vi "Main-revision3.vi"() -> ()   [LabVIEW 2013]
uses:
  Controls/GUI controls/TabControl--Tab.ctl
  Controls/Loop_data--Cluster.ctl
  Controls/Graph_data--Cluster.ctl
  Controls/GUI controls/GUI_Flags.ctl
  Shared/MySQL/typedefs/mysql_authentication.ctl
  Controls/Database Data.ctl
  Shared/MySQL/Preset Query Enum.ctl
  <userlib>/_OpenG.lib/array/array.llb/Filter 1D Array with Scalar (String)__ogtk.vi
panel:
  out "chnl data":string[](array[string])
  out "channels":string[](array[string])
  out "Selected Variables":string[][](array[string])=[["LB_EnergyMeter_1", "Reading.Channel 1", "Preamp [mJ]", "", "", ""], ["LB_EnergyMeter_2", "Reading.Channel 1", "Amplifier 2 [J]", "", "", ""], ["HPD_CCD", "exposure", "exposure", "0.003", "0.08", "0.0003"]]
  out "Device Infor from Database":string[][](array[string])
  out "subscribe messages\nfor Device status":string[](array[string])
  out "tcp Data":string[][](array[string])=[["LB_EnergyMeter_1 LB_EnergyMeter_1 shot #", "LB_EnergyMeter_1 reading.channel 1", "LB_EnergyMeter_2 LB_EnergyMeter_2 shot #", "LB_EnergyMeter_2 reading.channel 1", "HPD_CCD HPD_CCD shot #", "HPD_CCD exposure"], ["0", "0.029234726", "0", "0.000000000", "0", "0.003000"]]
  in  "Tab Control":enum32{"Home", "Settings", "Plot", "Save"}(tab)
  in  "Database Variable List":i32[](listbox)
  in  "Plotter ID (Simulate)":string
  out "Query":string
  in  "Add variables":bool
  out "Long Term Plot":cluster{timestamp[], dbl[]}[](graph)
  in  "Clear Graph":bool
  out "short Term Plot":cluster{timestamp[], dbl[]}[](graph) caption="Long Term Plot"
  in  "Stop":bool
  in  "Simulate":bool
  out "appargs 2":string[](array[string])
  out "min Left":i16
  out "min Top":i16
  out "max Right":i16
  out "max Bottom":i16
  in  "Read INI File":bool
  in  "Configuration File Path":path=path "C:/Users/Priyanka/Documents/Plotter/Data/Plot Configuration.txt"
  out "Subscribe commands":string[](array[string])=["Wait>>Exposure,Gain", "Wait>>Exposure"]
  out "appended array":string[][](array[string])
  in  "Plot":bool=TRUE
  in  "Settings":bool
  in  "Home":bool
  # "Settings"
  # "Plot"
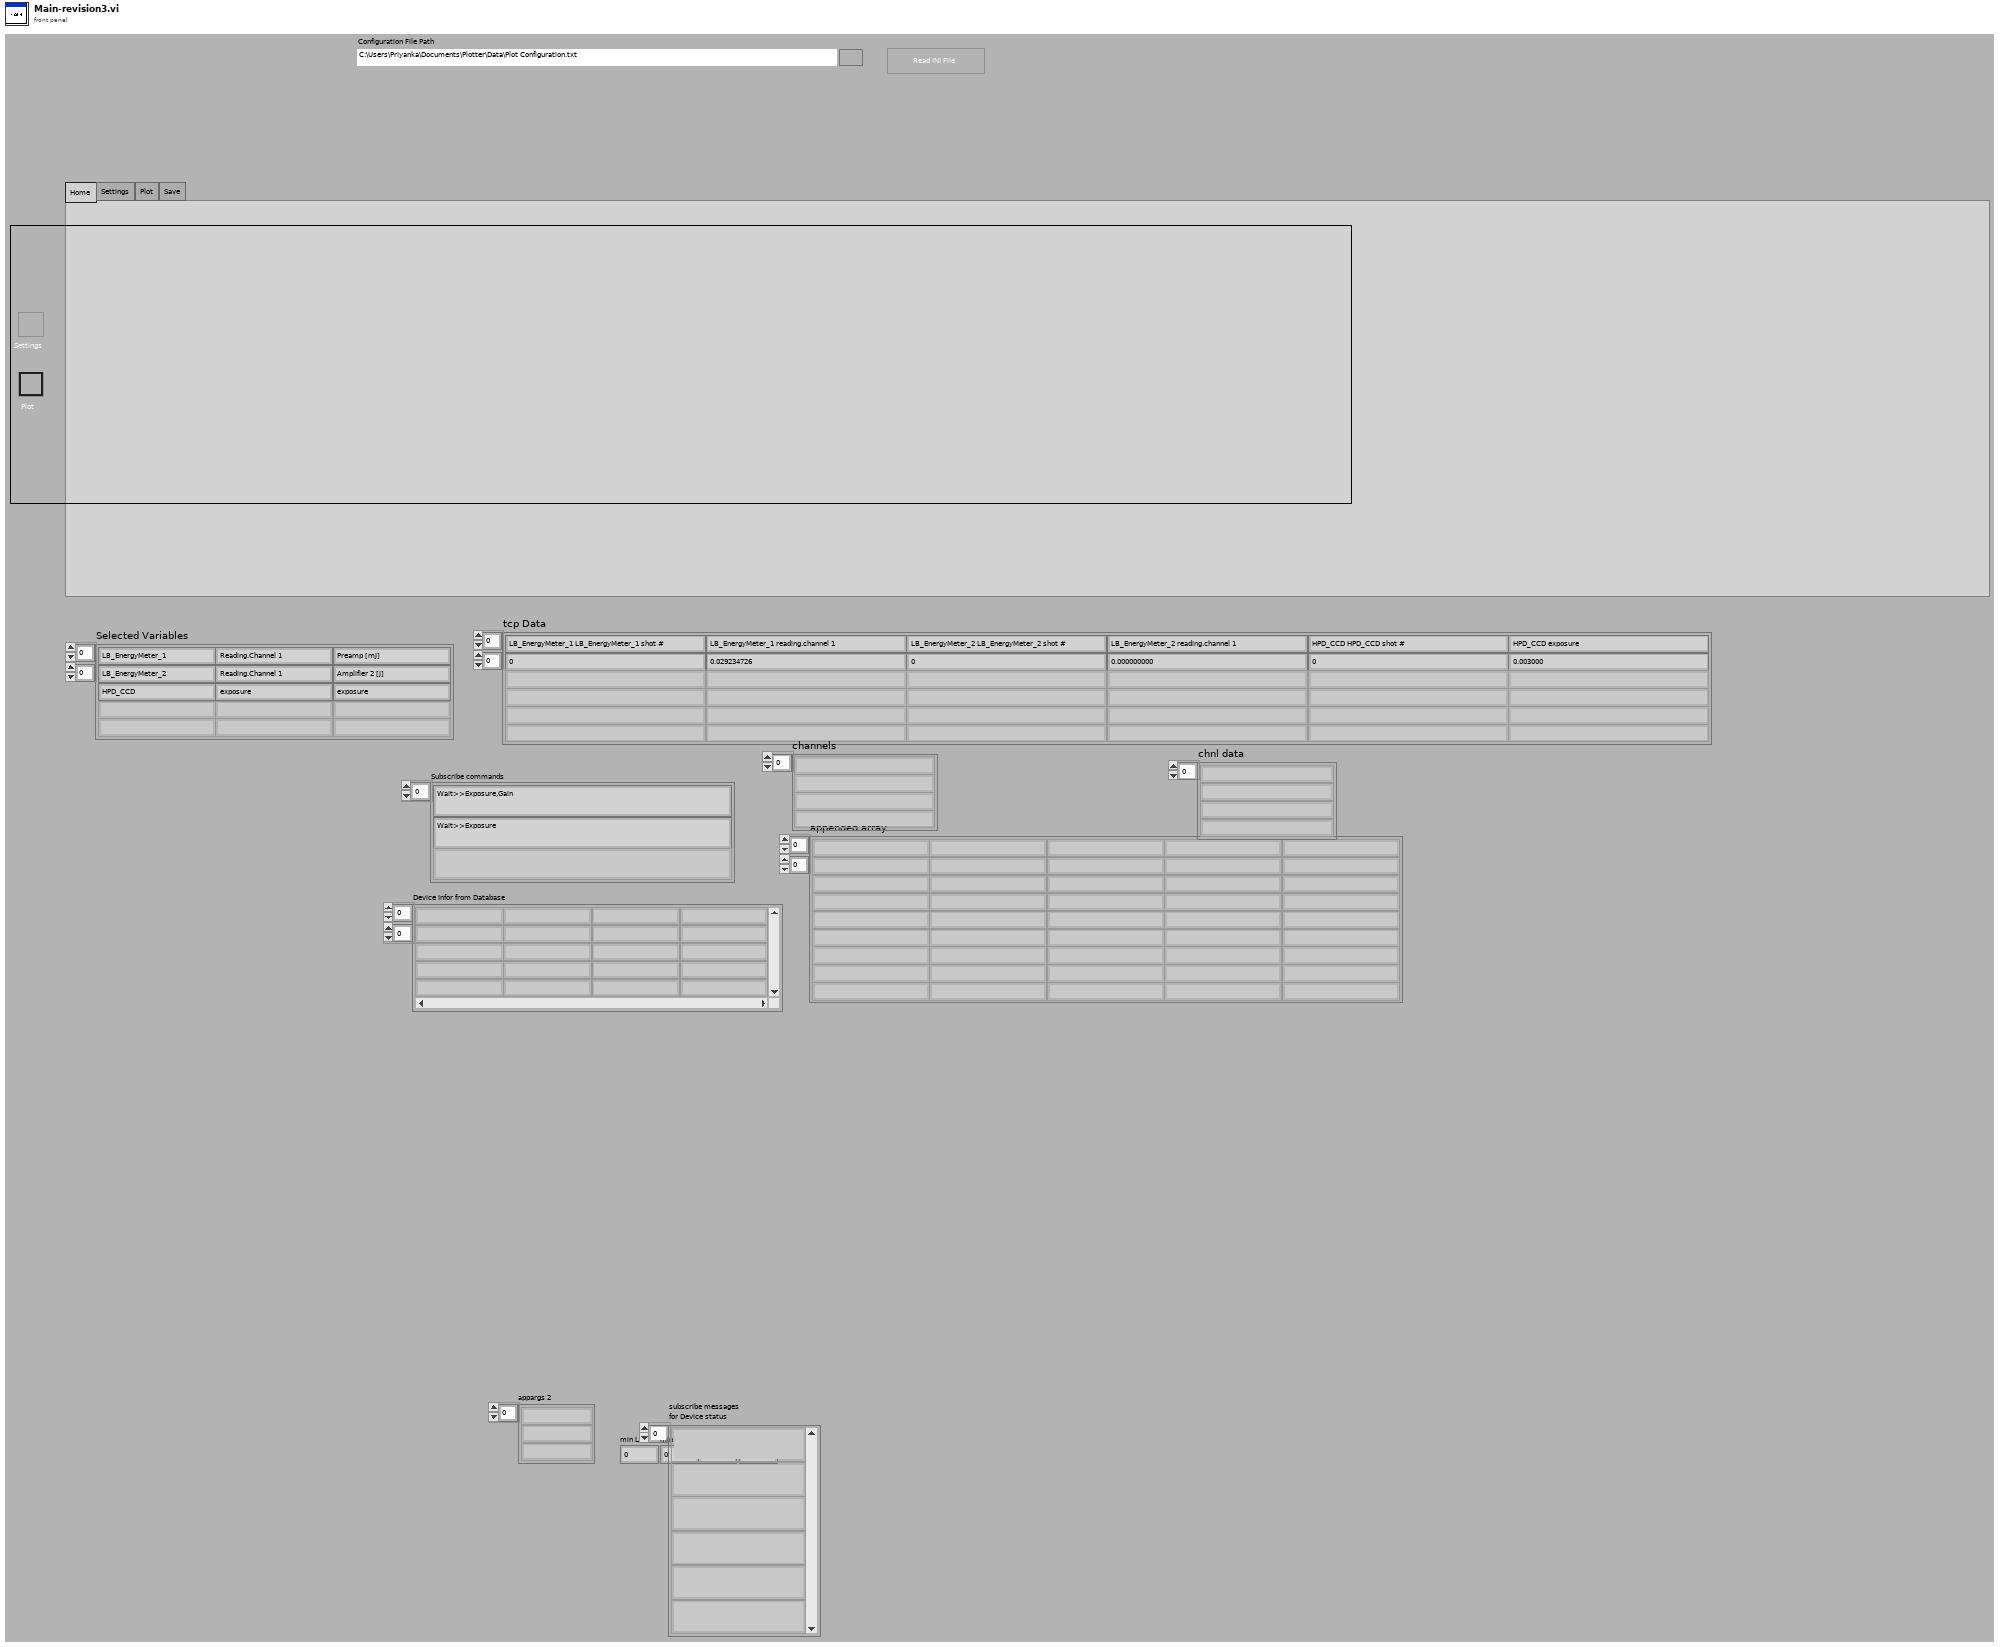
[diagram p1: front panel]
types:
  T1 = typedef "Preset Query Enum.ctl" = enum16{"Get Locations", "Get all IPs and MACs", "Get classes", "Get expt variables to set at scanstart for particular device", "Get expt devices and variables with start values", "Get expt devices and variables (with data to get)", "Get expt devices with data to get", "Get Expt devices and GUIs", "Get all devices basic properties", "Get Virtual Devices Core Info", "Get Expt names", "Get experiment basic properties", "Get experiment alarm variables", "Get MC Ports", "Get device network comm port", "Get devicetype lvclass path", "Get basic device properties", "Get Init Order", "Get all setable variables of a device", "Get device variable aliases", "Get force values of all settable variables", "Get all variables of a devicetype", "Get all variables of a device", "Get plotter details", "Get Saved Scans", "Get Scan Info", "GetGeneralGUIs", "Get expt for plotter", "Get plotter IDs from expt", "Get all devices", "Get all Virtual Devices", "Get all aliases", "Get variable and device info for Virtual Device", "GetItemLocatorIP", "Get IPs for GUIs", "Get DeviceType from Device", "GetLocalPortRange", "GetDevicePresetVariables", "Get Device Configuration", "GetAllPresetNames", "GetAllConfigurationNames", "GetPresetDeviceNames"}
  T2 = typedef "LVAllMonitorsDisplayTypeDef.ctl" = cluster{"Bounds":cluster{"Left":i16, "Top":i16, "Right":i16, "Bottom":i16}, "Depth":i16}[]
  T3 = typedef "tcp_new_data_event.ctl" = refnum<user-event>
  T4 = typedef "TabControl--Tab.ctl" = enum32{"Home", "Settings", "Plot", "Save"}
  T5 = enum32{"invalid app kind", "Development System", "Run Time System", "Student Edition", "Embedded LabVIEW", "Evaluation", "Custom"}
  T6 = enum32{"Invalid", "Standard", "Closed", "Hidden", "Minimized", "Maximized"}
  T7 = typedef "Loop_data--Cluster.ctl" = cluster{"INI Data":string[][], "Currently selected items":i32[], "Selected Variables":string[][], "No of Selected Variables":i32, "Data":dbl[], "Simulate":bool, "Start":bool, "Legend Rows":i32, "Init":bool}
  T8 = typedef "Graph_data--Cluster.ctl" = cluster{"Graph Data Long":cluster{"Timestamp":timestamp[], "Data Array":dbl[]}[], "Graph Data Short":cluster{"Timestamp":timestamp[], "Data Array":dbl[]}[], "Short term plot":refnum<vi>, "Long term plot ":refnum<vi>, "ms timer value":u32}
  T9 = typedef "GUI_Flags.ctl" = cluster{"Start":bool, "Stop":bool, "Read INI File":bool, "Tab Control":enum32{"Home", "Settings", "Plot", "Save"}, "Settings":bool, "Home":bool, "Plot":bool}
  T10 = typedef "Database Data.ctl" = cluster{"SQL Server Info":cluster{"Port":u16, "IP Address":string, "Authentication":T11}, "Variables":string[], "Devices":string[], "Display Names (for variables)":string[], "Variable Data ID":string, "Variable display info":string[][], "Plotter ID":string, "Device space Variable":string[]}
  T11 = typedef "mysql_authentication.ctl" = cluster{"User":string, "Password":string, "Database":string}
  T12 = cluster{"Core":cluster{"Current VI Reference":refnum<vi>, "Close Panel on Exit?":bool}, "Data":T7, "Graph":T8, "GUI controls":T9, "PlotterInfo (from DB)":T10, "Subscribe commands":string[]}
  T13 = cluster{"Current VI Reference":refnum<vi>, "Close Panel on Exit?":bool}
  T14 = cluster{"Port":u16, "IP Address":string, "Authentication":T11}
  T15 = cluster{"Timestamp":timestamp[], "Data Array":dbl[]}[]
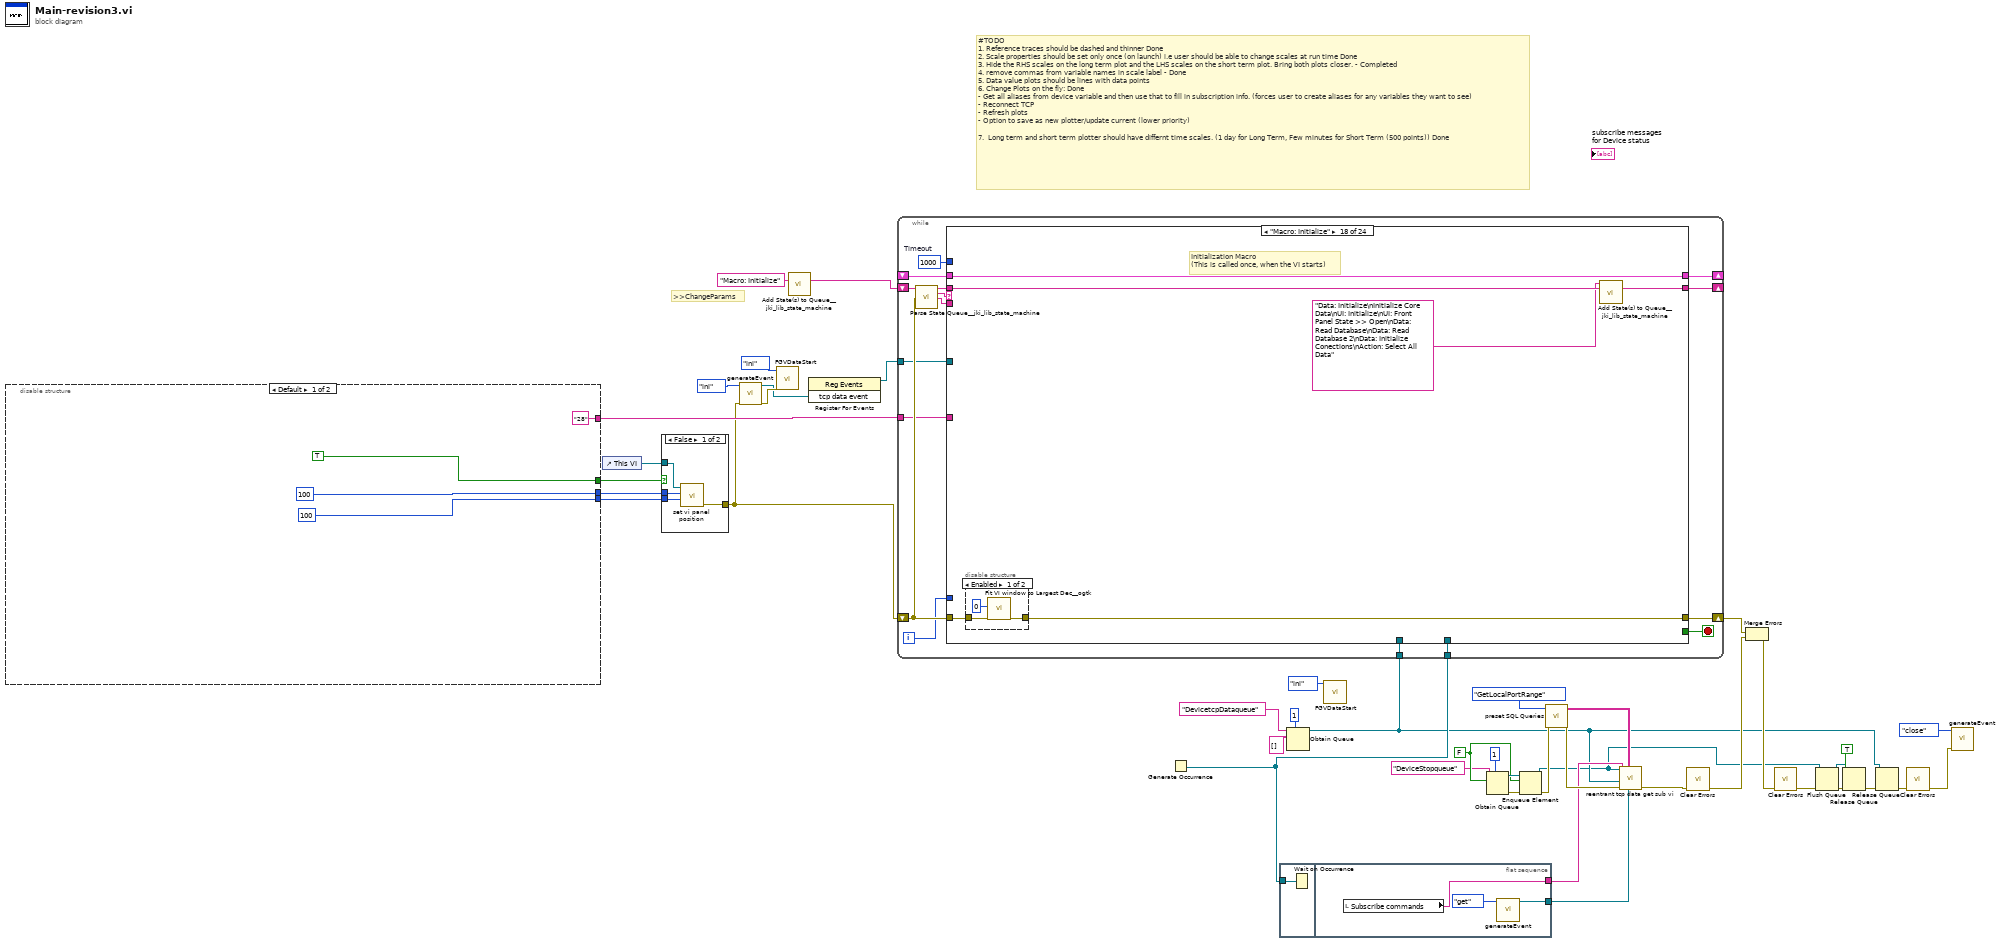
[diagram p0: block diagram]
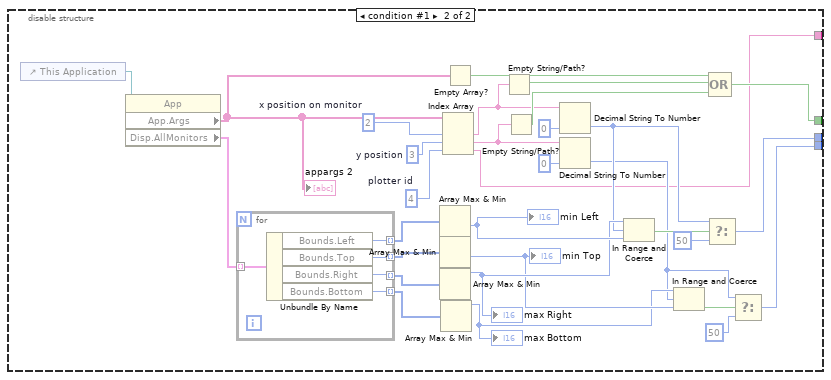
[diagram p3: hidden frame]
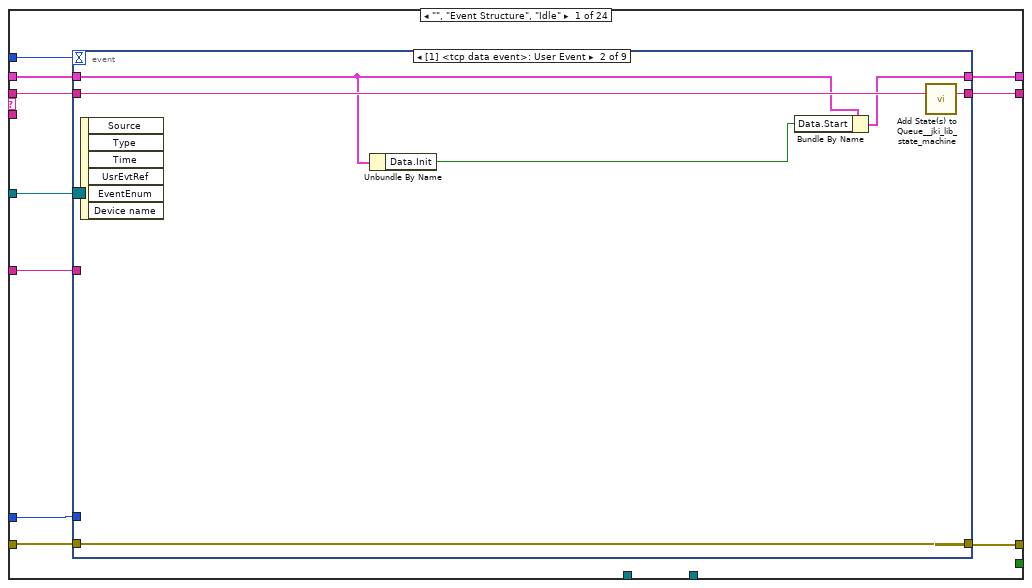
[diagram p4: hidden frame]
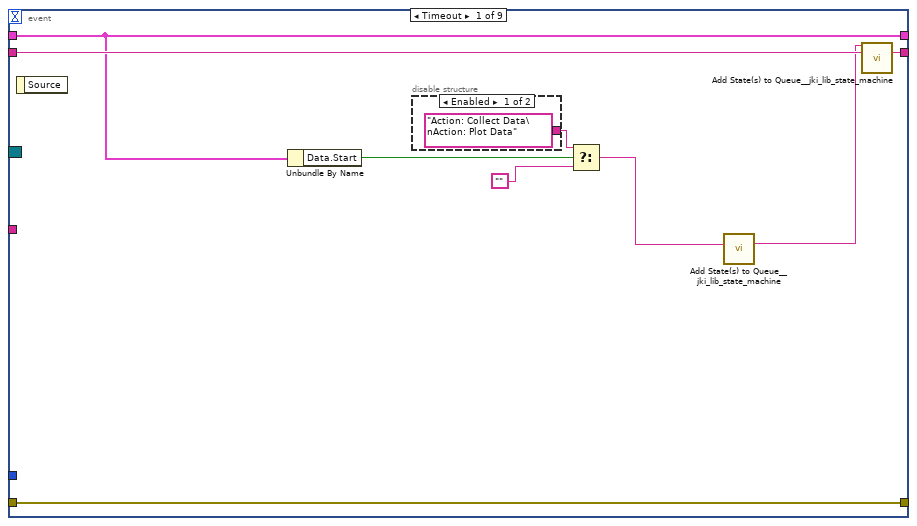
[diagram p5: hidden frame]
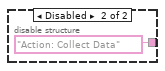
[diagram p6: hidden frame]
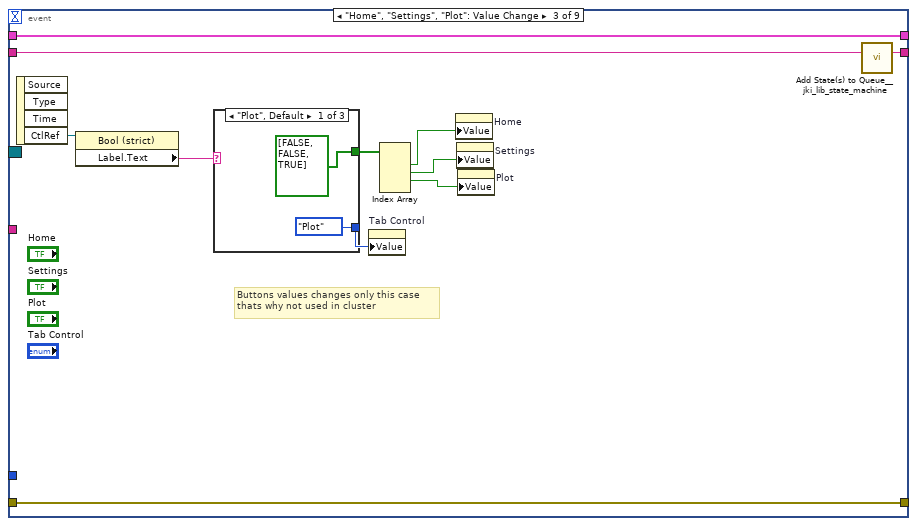
[diagram p7: hidden frame]
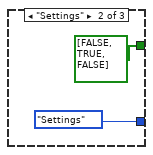
[diagram p8: hidden frame]
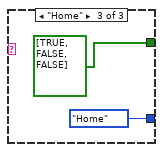
[diagram p9: hidden frame]
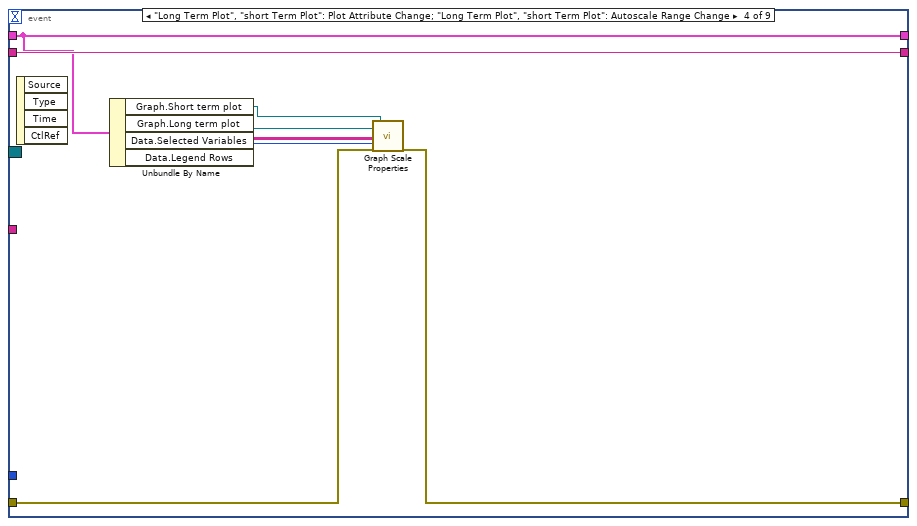
[diagram p10: hidden frame]
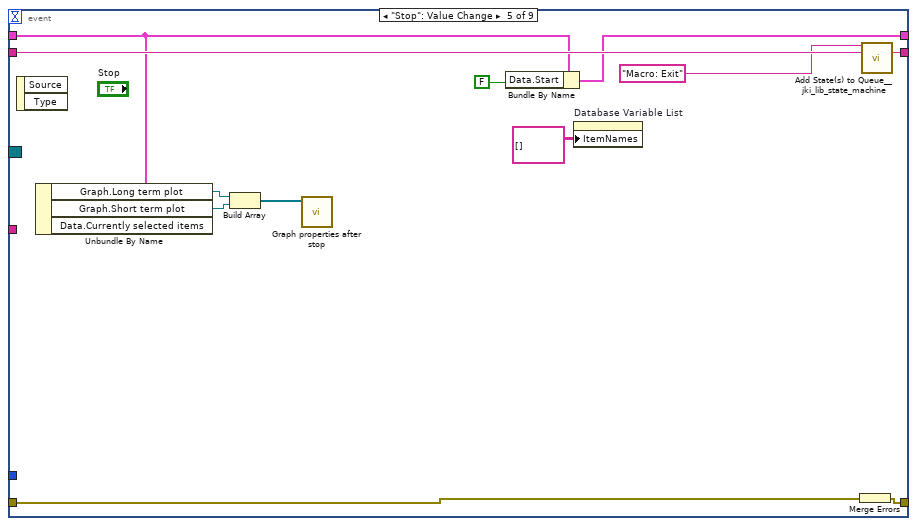
[diagram p11: hidden frame]
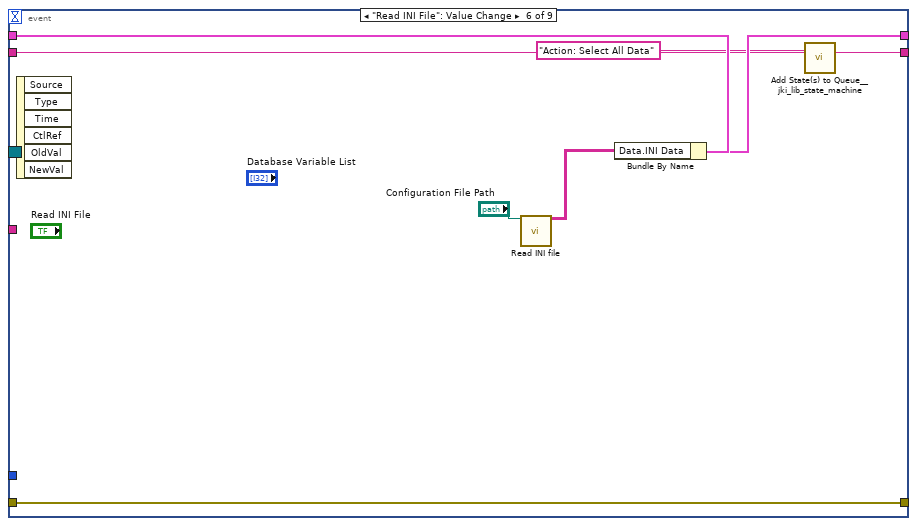
[diagram p12: hidden frame]
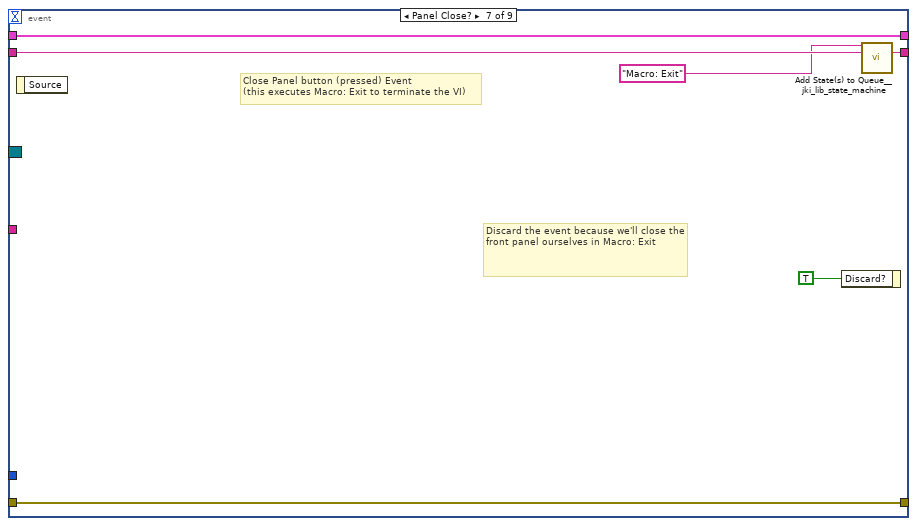
[diagram p13: hidden frame]
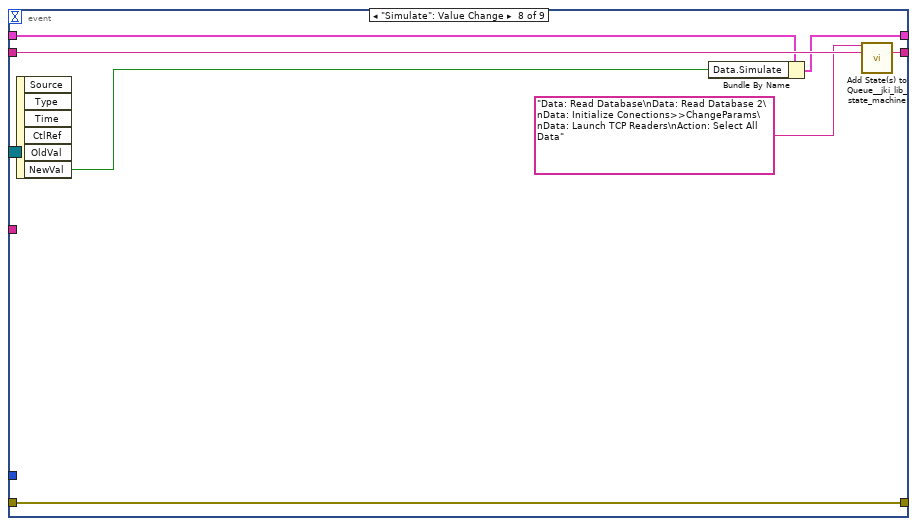
[diagram p14: hidden frame]
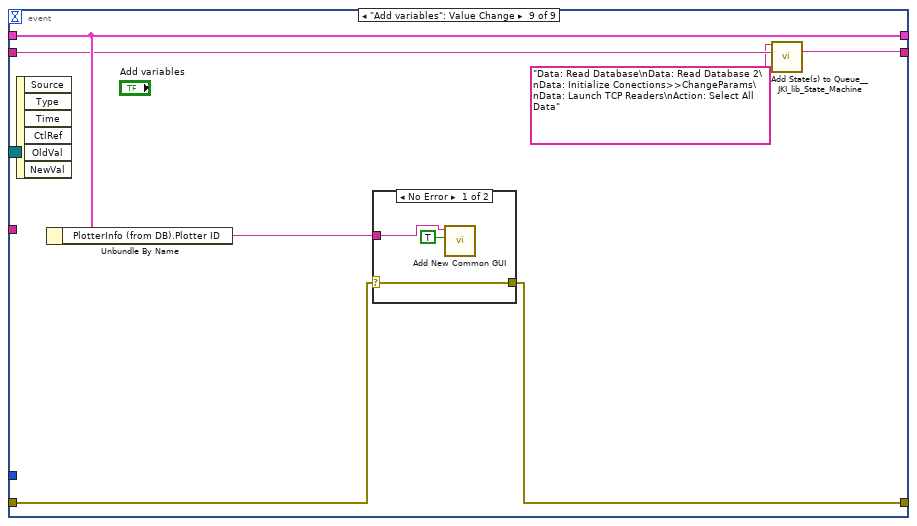
[diagram p15: hidden frame]
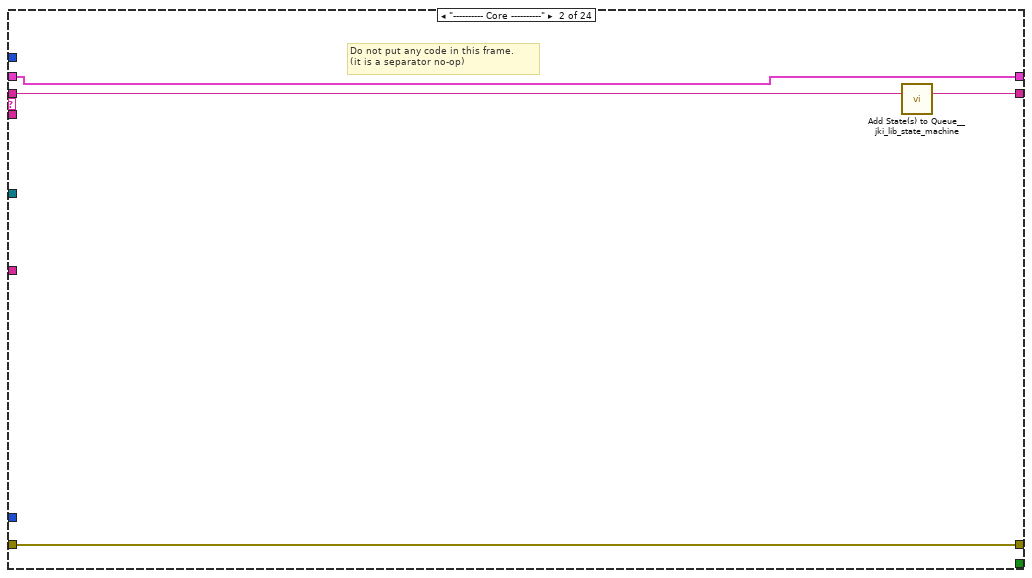
[diagram p17: hidden frame]
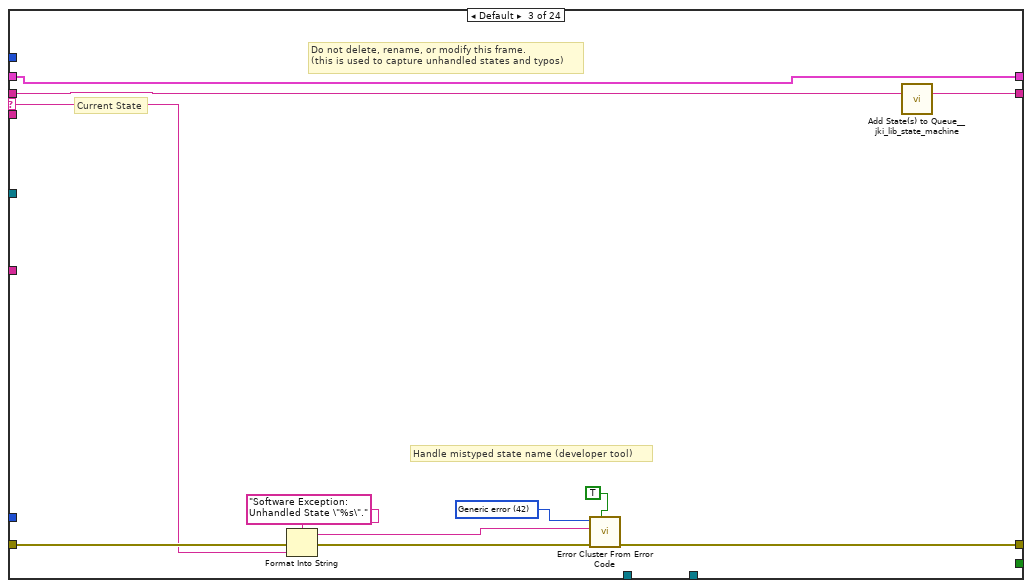
[diagram p18: hidden frame]
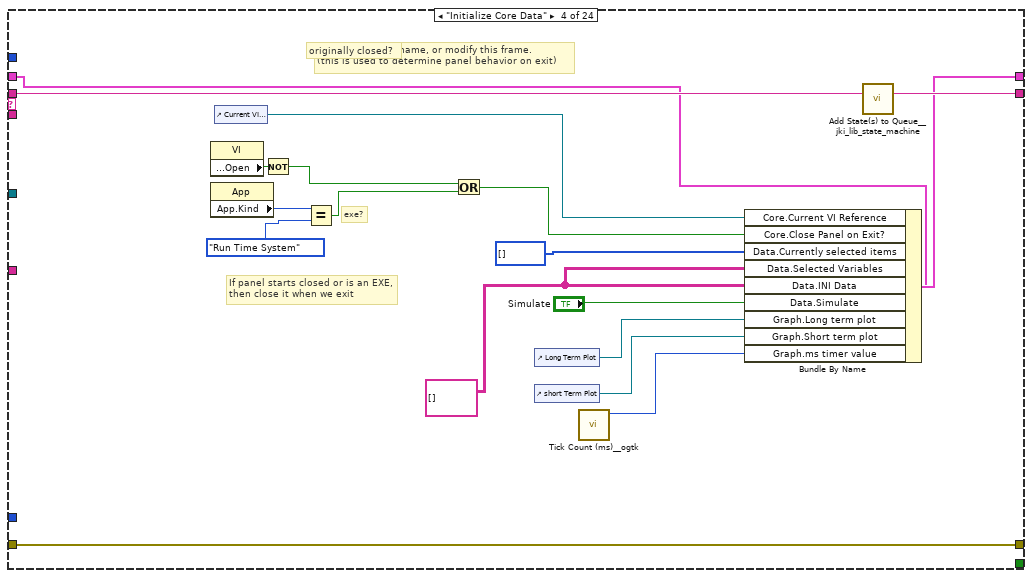
[diagram p19: hidden frame]
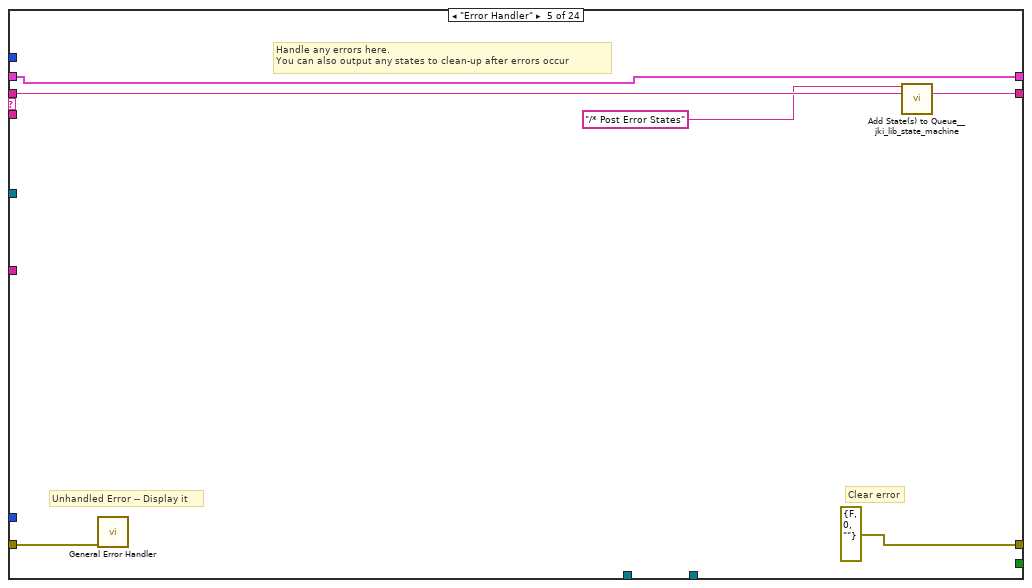
[diagram p20: hidden frame]
diagram:
  w23 = FALSE
  # ">>ChangeParams"
  # "#TODO\n1. Reference traces should be dashed and thinner Done\n2. Scale properties should be set only once (on launch) i.e user should be able to change scales at run time Done\n3. Hide the RHS scales on the long term plot and the LHS scales on the short term plot. Bring both plots closer. - Completed\n4. remove commas from variable names in scale label - Done \n5. Data value plots should be lines with data points\n6. Change Plots on the fly: Done\n- Get all aliases from device variable and then use that to fill in subscription info. (forces user to create aliases for any variables they want to see)\n- Reconnect TCP\n- Refresh plots\n- Option to save as new plotter/update current (lower priority)\n\n7.  Long term and short term plotter should have differnt time scales. (1 day for Long Term, Few minutes for Short Term (500 points)) Done"
  n1 = disable-structure shown="Default" {
    disable-tunnel: [100 ("number") w62] -> w39
    disable-tunnel: [100 ("number") w57] -> w40
    disable-tunnel: [TRUE w52] -> w41
    disable-tunnel: ["28" w49] -> w37
    frame condition #0 (active) {
    }
    frame condition #1 {
      w50 = 4  # plotter id
      w77 = 3  # y position
      w78 = 2  # x position on monitor
      n2 = control-ref of="This Application"() -> (w51:refnum<vi>)
      n3 = property class="App"(reference=w51) -> ("App.Args"=w76:string[], "Disp.AllMonitors"=w71:T2)  [unwired: 1 in, 2 out]
      "appargs 2" <- w76
      n4 = for {
        tunnel: w71 -> [w83] mode=indexing
        tunnel: [w82] -> w72 mode=indexing
        tunnel: [w81] -> w73 mode=indexing
        tunnel: [w80] -> w74 mode=indexing
        tunnel: [w79] -> w75 mode=indexing
        n5 = Unbundle By Name(w83) -> ("Bounds.Left"=w82:i16, "Bounds.Top"=w81:i16, "Bounds.Right"=w80:i16, "Bounds.Bottom"=w79:i16)
      }
      n6 = Array Max & Min(array=w72) -> (min value=w70:i16)  [unwired: 3 out]
      "min Left" <- w70
      n7 = Array Max & Min(array=w73) -> (min value=w68:i16)  [unwired: 3 out]
      "min Top" <- w68
      n8 = Array Max & Min(array=w74) -> (max value=w69:i16)  [unwired: 3 out]
      "max Right" <- w69
      n9 = Array Max & Min(array=w75) -> (max value=w67:i16)  [unwired: 3 out]
      "max Bottom" <- w67
      n10 = Index Array(array=w76, index #1=w78, index #2=w77, index #3=w50) -> (element #1=w48:string, element #2=w56:string, element #3=w49:string)
      n11 = Empty Array?(array=w76) -> (empty?=w55:bool)
      n12 = Empty String/Path?(string/path=w48) -> (empty?=w54:bool)
      n13 = Empty String/Path?(string/path=w56) -> (empty?=w53:bool)
      n14 = Decimal String To Number(string=w48, default (0L)=i16 0 ("default (0 I32)")) -> (number=w63:i16)  [unwired: 1 in, 1 out]
      n15 = Decimal String To Number(string=w56, default (0L)=i16 0 ("default (0 I32)")) -> (number=w58:i16)  [unwired: 1 in, 1 out]
      n16 = In Range and Coerce(upper limit=w69, x=w63, lower limit=w70) -> (In Range?=w64:bool)  [unwired: 1 out]
      n17 = In Range and Coerce(upper limit=w67, x=w58, lower limit=w68) -> (In Range?=w59:bool)  [unwired: 1 out]
      n18 = Select(t=w63, s=w64, f=i16 50) -> (s? t:f=w62:i16)
      n19 = Compound Arithmetic op=OR(w55, w54, w53) -> (w52:bool)
      n20 = Select(t=w58, s=w59, f=i16 50) -> (s? t:f=w57:i16)
    }
  }
  n21 = control-ref of="This VI"() -> (w38:refnum<vi>)
  n22 = case shown="False" w41 {
    tunnel: w39 -> [w87 _]
    tunnel: w40 -> [w86 _]
    tunnel: w38 -> [w85 _]
    tunnel: [w84 _] -> w6
    frame False {
      n23 = call "set vi panel position.vi"("top"=w86, "left"=w87, "This VI"=w85) -> ("error out"=w84:errorcluster)  [unwired: 7 in, 1 out]
    }
    frame True {
    }
  }
  n24 = call "generateEvent.vi"("error in"=w6, "command"=enum16{"ini", "get", "close"}."ini") -> ("error out"=w4:errorcluster, "tcp data event"=w2:T3)  [unwired: 8 in]
  n25 = call "FGVDataStart.vi"("error in"=w4, "command"=enum16{"ini", "get", "set"}."ini") -> ()  [unwired: 8 in, 2 out]
  n26 = call <vilib>:"Add State(s) to Queue__jki_lib_state_machine.vi"("State(s) in (\"\")"="Macro: Initialize") -> ("States Out"=w43:string)  [unwired: 14 in]
  n27 = register-events(w2) -> (reference out=w1:refnum<event-registration>)  [unwired: 2 in, 1 out]
  n28 = Generate Occurrence() -> (w15:refnum<k4>)
  n29 = flat-sequence {
    tunnel: w15 -> [w88]
    tunnel: [w89] -> w27
    tunnel: [w90] -> w28
    frame #0 {
      n30 = Wait on Occurrence(2:w88) -> ()  [unwired: 2 in, 1 out]
    }
    frame #1 {
      n31 = local read "Subscribe commands"() -> (w89:string[])
      n32 = call "generateEvent.vi"("command"=enum16{"ini", "get", "close"}."get") -> ("tcp data event"=w90:T3)  [unwired: 9 in, 1 out]
    }
  }
  n33 = Obtain Queue(max queue size (-1, unlimited)=1, name (unnamed)="DevicetcpDataqueue", element data type=string[][] [] ("Data in")) -> (queue out=w11:refnum<queue>)  [unwired: 2 in, 2 out]
  n34 = while {
    shift-right: [w101] -> _
    shift-left: _ -> [w100]
    shift-right: [w104] -> w14
    shift-left: w6 -> [w98]
    shift-right: [w103] -> _
    shift-left: w43 -> [w105]
    tunnel: w37 -> [w96]
    tunnel: w15 -> [w95]
    tunnel: w11 -> [w94]
    tunnel: w1 -> [w92]
    i -> [w93]
    stop <- w102 stop-if-true
    w99 = 1000  # Timeout
    n35 = call <vilib>:"Parse State Queue__jki_lib_state_machine.vi"("State Queue"=w105, "Error In (no error)"=w98) -> ("Remaining States"=w107:string, "Current State"=w97:string, "Arguments"=w106:string)  [unwired: 11 in]
    n36 = case shown="\"Macro: Initialize\"" w97 {
      selector: w97 -> [_ _ w208 _ _ _ _ _ _ _ _ _ _ _ _ _ _ _ _ _ _ _ _ _]
      tunnel: w107 -> [w117 w207 w212 w236 w242 w247 w251 w261 w267 w288 w325 w343 w370 w380 w386 w397 w423 w429 w449 w453 w457 w489 w514 w567]
      tunnel: w106 -> [_ _ _ _ _ _ _ _ _ _ _ _ _ _ w381 w391 _ _ _ _ _ _ _ _]
      tunnel: w100 -> [w115 w204 w210 w227 w239 w245 w248 _ w263 w275 w319 w340 w367 w371 w384 w393 w420 w425 w446 w450 w459 w484 w509 w563]
      tunnel: [w114 w205 w214 w233 errorcluster {"status"=FALSE, "code"=0, "source"=""} ("error out") w244 w249 w258 w262 w286 w322 w336 w368 w378 w382 w394 w421 w426 w447 w451 w465 w487 w510 w559] -> w104
      tunnel: w98 -> [w113 w205 w213 w233 w238 w244 w249 w258 w264 w286 w323 w337 w368 w378 w383 w395 w421 w427 w447 w451 w465 w487 w511 w551]
      tunnel: [w116 w206 w211 w235 w241 w246 w250 w260 w266 w287 w324 w342 w369 w379 w385 w396 w422 w428 w448 w452 w456 w488 w513 w566] -> w103
      tunnel: [_ _ _ _ _ TRUE _ _ _ _ _ _ _ _ _ _ _ _ _ _ _ _ _ _] -> w102
      tunnel: [w112 w204 w210 w234 w239 w245 w248 w259 w263 w285 w321 w339 w367 w371 w384 w393 w420 w425 w446 w450 w458 w485 w508 w565] -> w101
      tunnel: w99 -> [w111 _ _ _ _ _ _ _ _ _ _ _ _ _ _ _ _ _ _ _ _ _ _ _]
      tunnel: w96 -> [w110 _ _ _ _ _ _ _ _ w272 _ _ _ _ _ _ _ _ _ _ _ _ _ _]
      tunnel: w95 -> [_ _ _ _ _ _ _ _ _ _ _ w332 _ _ _ _ _ _ _ _ _ _ _ _]
      tunnel: w94 -> [_ _ _ _ _ _ _ _ _ _ _ _ _ _ _ _ _ _ _ _ _ _ w505 _]
      tunnel: w93 -> [w109 _ _ _ _ _ _ _ _ _ _ _ _ _ _ _ _ _ _ _ _ _ _ _]
      tunnel: w92 -> [w108 _ _ _ _ _ _ _ _ _ _ _ _ _ _ _ _ _ _ _ _ _ _ _]
      frame "", "Event Structure", "Idle" {
        n37 = event shown="[1] <tcp data event>: User Event" {
          selector: w108 -> [_ _ _ _ _ _ _ _ _]
          dyn-events: _ -> [_ _ _ _ _ _ _ _ _]
          timeout: w111 -> [_ _ _ _ _ _ _ _ _]
          tunnel: w117 -> [w126 w134 w145 w159 w171 w174 w185 w192 w197]
          tunnel: [w125 w133 w144 w159 w170 w173 w184 w191 w196] -> w116
          tunnel: w115 -> [w123 w130 w139 w158 w165 w176 w182 w189 w199]
          tunnel: [w124 w132 w143 w154 w160 w179 w183 w190 w193] -> w114
          tunnel: w113 -> [w124 w132 w143 w155 w169 w179 w183 w190 w194]
          tunnel: [w123 w131 w139 w158 w167 w175 w182 w188 w199] -> w112
          tunnel: w110 -> [_ _ _ _ _ _ _ _ _]
          tunnel: w109 -> [_ _ _ _ _ _ _ _ _]
          event Timeout {
            n38 = event-data() -> ()  [unwired: 1 in, 1 out]
            n39 = Unbundle By Name(w123) -> ("Data.Start"=w119:bool)
            n40 = disable-structure shown="Enabled" {
              disable-tunnel: ["Action: Collect Data\nAction: Plot Data" ("f") "Action: Collect Data" ("f")] -> w122
              frame Enabled {
              }
              frame Disabled {
              }
            }
            n41 = Select(t=w122, s=w119, f="") -> (s? t:f=w120:string)
            n42 = call <vilib>:"Add State(s) to Queue__jki_lib_state_machine.vi"("State(s) in (\"\")"=w120) -> ("States Out"=w118:string)  [unwired: 14 in]
            n43 = call <vilib>:"Add State(s) to Queue__jki_lib_state_machine.vi"("State(s) in Front (\"\")"=w118, "State(s) in (\"\")"=w126) -> ("States Out"=w125:string)  [unwired: 13 in]
          }
          event User Event {
            n44 = event-data() -> ()  [unwired: 1 in, 6 out]
            n45 = Unbundle By Name(w130) -> ("Data.Init"=w129:bool)
            n46 = Bundle By Name(cluster=w130, "Data.Start"=w129) -> (w131:T12)
            n47 = call <vilib>:"Add State(s) to Queue__jki_lib_state_machine.vi"("State(s) in (\"\")"=w134) -> ("States Out"=w133:string)  [unwired: 14 in]
          }
          event "Home", "Settings", "Plot": Value Change {
            # "Buttons values changes only this case \nthats why not used in cluster"
            n48 = event-data() -> ("CtlRef"=w142:refnum<vi>)  [unwired: 1 in, 3 out]
            n49 = property class="Bool (strict)"(reference=w142) -> ("Label.Text"=w141:string)  [unwired: 1 in, 2 out]
            n50 = case shown="\"Plot\", Default" w141 {
              tunnel: [TabControl--Tab."Plot" ("Tab Control") TabControl--Tab."Settings" ("Tab Control") TabControl--Tab."Home" ("Tab Control")] -> w135
              tunnel: [bool[] [FALSE, FALSE, TRUE] bool[] [FALSE, TRUE, FALSE] bool[] [TRUE, FALSE, FALSE]] -> w140
              frame "Plot", Default {
              }
              frame "Settings" {
              }
              frame "Home" {
              }
            }
            n51 = property on="Tab Control" class="TabCtl (strict)"("Value"=w135) -> ()  [unwired: 2 in, 2 out]
            n52 = Index Array(array=w140) -> (element #1=w138:bool, element #2=w137:bool, element #3=w136:bool)  [unwired: 4 in, 1 out]
            n53 = property on="Home" class="Bool (strict)"("Value"=w138) -> ()  [unwired: 2 in, 2 out]
            n54 = property on="Settings" class="Bool (strict)"("Value"=w137) -> ()  [unwired: 2 in, 2 out]
            n55 = property on="Plot" class="Bool (strict)"("Value"=w136) -> ()  [unwired: 2 in, 2 out]
            n56 = call <vilib>:"Add State(s) to Queue__jki_lib_state_machine.vi"("State(s) in (\"\")"=w145) -> ("States Out"=w144:string)  [unwired: 14 in]
          }
          event "Long Term Plot", "short Term Plot": Plot Attribute Change; "Long Term Plot", "short Term Plot": Autoscale Range Change {
            n57 = event-data() -> ()  [unwired: 1 in, 4 out]
            n58 = Unbundle By Name(w158) -> ("Graph.Short term plot"=w156:refnum<vi>, "Graph.Long term plot"=w152:refnum<vi>, "Data.Selected Variables"=w157:string[][], "Data.Legend Rows"=w153:i32)
            n59 = call "Graph Scale Properties.vi"("Long term plot"=w152, "Selected Variables"=w157, "Legend Rows"=w153, "error in (no error)"=w155, "Short term graph"=w156) -> ("error out"=w154:errorcluster)  [unwired: 14 in]
          }
          event "Stop": Value Change {
            n60 = event-data() -> ()  [unwired: 1 in, 2 out]
            n61 = Unbundle By Name(w165) -> ("Graph.Long term plot"=w162:refnum<vi>, "Graph.Short term plot"=w161:refnum<vi>)  [unwired: 1 out]
            n62 = Build Array(w162, w161) -> (w163:refnum<vi>[])
            n63 = call "Graph properties after stop.vi"("Array"=w163) -> ()  [unwired: 11 in]
            n64 = Bundle By Name(cluster=w165, "Data.Start"=FALSE) -> (w167:T12)
            n65 = property on="Database Variable List" class="MCListbox (strict)"("ItemNames"=string[][] [] ("Item Names")) -> ()  [unwired: 2 in, 2 out]
            n66 = Merge Errors(w169) -> (w160:errorcluster)
            n67 = call <vilib>:"Add State(s) to Queue__jki_lib_state_machine.vi"("State(s) in Front (\"\")"="Macro: Exit", "State(s) in (\"\")"=w171) -> ("States Out"=w170:string)  [unwired: 13 in]
          }
          event "Read INI File": Value Change {
            n68 = event-data() -> ()  [unwired: 1 in, 6 out]
            n69 = call "Read INI file.vi"("Path"="Configuration File Path") -> ("Data"=w177:string[][])  [unwired: 9 in, 5 out]
            n70 = Bundle By Name(cluster=w176, "Data.INI Data"=w177) -> (w175:T12)
            n71 = call <vilib>:"Add State(s) to Queue__jki_lib_state_machine.vi"("State(s) in Front (\"\")"="Action: Select All Data" ("State(s) in Front (\"\")"), "State(s) in (\"\")"=w174) -> ("States Out"=w173:string)  [unwired: 13 in]
          }
          event Panel Close? {
            # "Discard the event because we'll close the front panel ourselves in Macro: Exit"
            # "Close Panel button (pressed) Event\n(this executes Macro: Exit to terminate the VI)"
            n72 = event-data() -> ()  [unwired: 1 in, 1 out]
            n73 = event-data("Discard?"=TRUE) -> ()  [unwired: 1 in, 1 out]
            n74 = call <vilib>:"Add State(s) to Queue__jki_lib_state_machine.vi"("State(s) in Front (\"\")"="Macro: Exit", "State(s) in (\"\")"=w185) -> ("States Out"=w184:string)  [unwired: 13 in]
          }
          event "Simulate": Value Change {
            n75 = event-data() -> ("NewVal"=w187:bool)  [unwired: 1 in, 5 out]
            n76 = Bundle By Name(cluster=w189, "Data.Simulate"=w187) -> (w188:T12)
            n77 = call <vilib>:"Add State(s) to Queue__jki_lib_state_machine.vi"("State(s) in Front (\"\")"="Data: Read Database\nData: Read Database 2\nData: Initialize Conections>>ChangeParams\nData: Launch TCP Readers\nAction: Select All Data" ("State(s) in Front (\"\")"), "State(s) in (\"\")"=w192) -> ("States Out"=w191:string)  [unwired: 13 in]
          }
          event "Add variables": Value Change {
            n78 = event-data() -> ()  [unwired: 1 in, 6 out]
            n79 = Unbundle By Name(w199) -> ("PlotterInfo (from DB).Plotter ID"=w198:string)
            n80 = case shown="No Error" w194 {
              selector: w194 -> [w200 w203]
              tunnel: w198 -> [w201 _]
              tunnel: [w200 w203] -> w193
              frame No Error {
                n81 = call "Add New Common GUI.vi"("With Alias"=TRUE, "Plotter ID"=w201) -> ()  [unwired: 10 in]
              }
              frame Error {
              }
            }
            n82 = call <vilib>:"Add State(s) to Queue__JKI_lib_State_Machine.vi"("State(s) in Front (\"\")"="Data: Read Database\nData: Read Database 2\nData: Initialize Conections>>ChangeParams\nData: Launch TCP Readers\nAction: Select All Data", "State(s) in (\"\")"=w197) -> ("States Out"=w196:string)  [unwired: 13 in]
          }
        }
      }
      frame "---------- Core ----------" {
        # "Do not put any code in this frame.\n(it is a separator no-op)"
        n83 = call <vilib>:"Add State(s) to Queue__jki_lib_state_machine.vi"("State(s) in (\"\")"=w207) -> ("States Out"=w206:string)  [unwired: 14 in]
      }
      frame Default {
        w217 = 42 items=["No error", "Argument error", "Memory is full", "Out of zone", "End of file", "File already open", "Generic file I/O error", "File not found", "File permission error", "Disk is full", "Duplicate path", "Too many files open", "System feature not enabled", "Resource file not found", "Cannot add resource", "Resource not found", "Image not found", "Image memory error", "Pen does not exist", "Config type invalid", "Config token not found", "Config parse error", "Config memory error", "Bad external code format", "Bad external code offset", "External code not present", "Null window", "Destroy window error", "Null menu", "Print aborted", "Bad print record", "Print driver error", "Windows error during printing", "Memory error during printing", "Print dialog error", "Generic print error", "Invalid device refnum", "Device not found", "Device parameter error", "Device unit error", "Cannot open device", "Device call aborted", "Generic error", "Cancelled by user", "Object ID too low", "Object ID too high", "Object not in heap", "Unknown heap", "Unknown object (invalid DefProc)", "Unknown object (DefProc not in table)", "Message out of range", "Invalid (null) method", "Unknown message", "Manager call not supported", "Bad address", "Network operation in progress", "Network operation timed out", "Connection is busy", "Network attribute not supported", "Network error", "Address in use", "System out of memory", "Connection aborted", "Connection refused", "Not connected", "Already connected", "Connection closed", "Initialization error (interapplication manager)", "Bad occurrence", "Wait on unbound occurrence handler", "Occurrence queue overflow", "Datalog type conflict", "Unused", "Unrecognized type (interapplication manager)", "Memory corrupt", "Failed to make temporary DLL", "Old CIN version", "Drag socket not found", "Failed to load drop-object", "Failed to register OLE object", "Failed to release OLE object", "Format specifier type mismatch", "Unknown format specifier", "Too few format specifiers", "Too many format specifiers", "Scan failed", "Newer CIN version", "Error converting to variant", "Runtime menu error", "Password tampered", "Variant attribute not found", "Incompatible variant data type", "Event data is not available", "Event Store is not present", "Occurrence is not found", "Event Queue is not created", "Event info is not available", "Refnum passed is NULL", "Error retrieving Class GUID", "Error retrieving CoClass GUID", "Error retrieving TypeLib GUID.", "Bad built application magic bytes.", "Specific driver is different from the specific driver associated with the Logical Name.", "There is no session opened to the class driver.", "Max Error", "MAX - Error with config objects", "MAX - Error loading configuration", "MAX - Group not supported"]
        # "Current State"
        # "Do not delete, rename, or modify this frame.\n(this is used to capture unhandled states and typos)"
        # "Handle mistyped state name (developer tool)"
        n84 = Format Into String(format string="Software Exception: Unhandled State \"%s\"." ("message"), error in=w213, w208) -> (resulting string=w216:string, error out=w215:errorcluster)  [unwired: 1 in]
        n85 = call <vilib>:"Error Cluster From Error Code.vi"("show call chain? (False)"=TRUE, "error in (no error)"=w215, "error message (\"\")"=w216, "error code (0)"=w217) -> ("error out"=w214:errorcluster)  [unwired: 5 in]
        n86 = call <vilib>:"Add State(s) to Queue__jki_lib_state_machine.vi"("State(s) in (\"\")"=w212) -> ("States Out"=w211:string)  [unwired: 14 in]
      }
      frame "Initialize Core Data" {
        w219 = string[][] [] ("Selected Variables")
        # "Do not delete, rename, or modify this frame.\n(this is used to determine panel behavior on exit)"
        # "originally closed?"
        # "exe?"
        # "If panel starts closed or is an EXE, then close it when we exit"
        n87 = property class="VI"() -> ("Front Panel.Open"=w232:bool)  [unwired: 2 in, 2 out]
        n88 = property class="App"() -> ("App.Kind"=w231:T5)  [unwired: 2 in, 2 out]
        n89 = control-ref of="Current VI Reference"() -> (w225:refnum<vi>)
        n90 = Not(x=w232) -> (.not. x?=w229:bool)
        n91 = Equal?(x=w231, y=T5."Run Time System" ("Application:Kind")) -> (x = y?=w228:bool)
        n92 = Or(x=w229, y=w228) -> (x .or. y?=w226:bool)
        n93 = control-ref of="Long Term Plot"() -> (w222:refnum<vi>)
        n94 = control-ref of="short Term Plot"() -> (w221:refnum<vi>)
        n95 = call <userlib>:"Tick Count (ms)__ogtk.vi"() -> ("millisecond timer value"=w220:u32)  [unwired: 10 in, 1 out]
        n96 = Bundle By Name(cluster=w227, "Core.Current VI Reference"=w225, "Core.Close Panel on Exit?"=w226, "Data.Currently selected items"=i32[] [], "Data.Selected Variables"=w219, "Data.INI Data"=w219, "Data.Simulate"="Simulate", "Graph.Long term plot"=w222, "Graph.Short term plot"=w221, "Graph.ms timer value"=w220) -> (w234:T12)
        n97 = call <vilib>:"Add State(s) to Queue__jki_lib_state_machine.vi"("State(s) in (\"\")"=w236) -> ("States Out"=w235:string)  [unwired: 14 in]
      }
      frame "Error Handler" {
        # "Unhandled Error -- Display it"
        # "Handle any errors here.\nYou can also output any states to clean-up after errors occur"
        # "Clear error"
        n98 = call <vilib>:"General Error Handler.vi"("error in (no error)"=w238) -> ()  [unwired: 10 in, 5 out]
        n99 = call <vilib>:"Add State(s) to Queue__jki_lib_state_machine.vi"("State(s) in Front (\"\")"="/* Post Error States", "State(s) in (\"\")"=w242) -> ("States Out"=w241:string)  [unwired: 13 in]
      }
      frame "Exit" {
        # "Do not put any code in this frame.\n(No errors that occur here will be handled.)"
        n100 = call <vilib>:"Add State(s) to Queue__jki_lib_state_machine.vi"("State(s) in (\"\")"=w247) -> ("States Out"=w246:string)  [unwired: 14 in]
      }
      frame "---------- Data ----------" {
        # "Do not put any code in this frame.\n(It is a separator no-op. You can make a copy of this frame to create a new Data frame)"
        n101 = call <vilib>:"Add State(s) to Queue__jki_lib_state_machine.vi"("State(s) in (\"\")"=w251) -> ("States Out"=w250:string)  [unwired: 14 in]
      }
      frame "Data: Initialize" {
        w252 = string[] []  # Subscribe commands
        w253 = T10 {"SQL Server Info"={"Port"=0, "IP Address"="", "Authentication"={"User"="", "Password"="", "Database"=""}}, "Variables"=[], "Devices"=[], "Display Names (for variables)"=[], "Variable Data ID"="", "Variable display info"=[], "Plotter ID"="", "Device space Variable"=[]}  # PlotterInfo (from DB)
        w254 = T9 {"Start"=FALSE, "Stop"=TRUE, "Read INI File"=TRUE, "Tab Control"=enum."Plot", "Settings"=FALSE, "Home"=FALSE, "Plot"=TRUE}  # GUI controls
        w255 = T8 {"Graph Data Long"=[], "Graph Data Short"=[], "Short term plot"=refnum, "Long term plot "=refnum, "ms timer value"=0}  # Graph
        w256 = T7 {"INI Data"=[], "Currently selected items"=[], "Selected Variables"=[], "No of Selected Variables"=0, "Data"=[], "Simulate"=FALSE, "Start"=FALSE, "Legend Rows"=0, "Init"=FALSE}  # Data
        w257 = T13 {"Current VI Reference"=refnum, "Close Panel on Exit?"=FALSE}  # Core
        n102 = Bundle("Core"=w257, "Data"=w256, "Graph"=w255, "GUI controls"=w254, "PlotterInfo (from DB)"=w253, "Subscribe commands"=w252) -> (w259:T12)  [unwired: 1 in]
        n103 = call <vilib>:"Add State(s) to Queue__jki_lib_state_machine.vi"("State(s) in (\"\")"=w261) -> ("States Out"=w260:string)  [unwired: 14 in]
      }
      frame "Data: Cleanup" {
        # "Cleanup any data and references, here. (this is  automatically, by the Macro: Exit)"
        n104 = Unbundle By Name(w263) -> ("Core.Current VI Reference"=w265:refnum<vi>)
        n105 = Close Reference(reference=w265, error in (no error)=w264) -> (error out=w262:errorcluster)
        n106 = call <vilib>:"Add State(s) to Queue__jki_lib_state_machine.vi"("State(s) in (\"\")"=w267) -> ("States Out"=w266:string)  [unwired: 14 in]
      }
      frame "Data: Read Database" {
        w278 = 0 ("disabled index (col)")
        # "Get Device, Variable Names and Display Names from commongui Table"
        n107 = Unbundle By Name(w275) -> ("Data.Simulate"=w274:bool)
        n108 = Select(t="Plotter ID (Simulate)", s=w274, f=w272) -> (s? t:f=w271:string)
        n109 = Concatenate Strings("SELECT variablesid FROM commongui WHERE id ='", w271, "'" ("string")) -> (w279:string)
        "Query" <- w279
        n110 = call "SQL Server Info.vi"() -> ("SQL Server Info"=w284:T14)
        n111 = call "SQL Query.vi"("error in (no error)"=w286, "SQL Server Info"=w284, "Query"=w279) -> ("data"=w277:string[][])  [unwired: 7 in, 1 out]
        n112 = Empty Array?(array=w277) -> (empty?=w276:bool)
        n113 = case shown="True" w276 {
          tunnel: w271 -> [_ w293]
          frame False {
          }
          frame True {
            n114 = Concatenate Strings("Please Check Plotter ID [" ("string"), w293, "] Plotter ID should match with id from commongui Table in Database." ("message")) -> (w294:string)
            n115 = One Button Dialog(message=w294, button name ("OK")="OK") -> ()  [unwired: 1 out]
          }
        }
        n116 = Index Array(array=w277, index (row)=w278, index (col)=w278) -> (element=w283:string)
        n117 = call "Get Device List.vi"("SQL Server Info"=w284, "userID"=w283) -> ("Display Names"=w282:string[], "Variables"=w269:string[], "Devices"=w270:string[])  [unwired: 7 in]
        n118 = for {
          tunnel: w270 -> [w291] mode=indexing
          tunnel: w269 -> [w292] mode=indexing
          tunnel: [w289] -> w268 mode=indexing
          n119 = call <vilib>:"Space Constant.vi"() -> ("String"=w290:string)
          n120 = Concatenate Strings(w291, w290, w292) -> (w289:string)
        }
        n121 = Bundle By Name(cluster=w275, "PlotterInfo (from DB).SQL Server Info"=w284, "PlotterInfo (from DB).Variable Data ID"=w283, "PlotterInfo (from DB).Devices"=w270, "PlotterInfo (from DB).Variables"=w269, "PlotterInfo (from DB).Display Names (for variables)"=w282, "PlotterInfo (from DB).Device space Variable"=w268, "PlotterInfo (from DB).Plotter ID"=w271) -> (w285:T12)
        n122 = call <vilib>:"Add State(s) to Queue__jki_lib_state_machine.vi"("State(s) in (\"\")"=w288) -> ("States Out"=w287:string)  [unwired: 14 in]
      }
      frame "Data: Read Database 2" {
        # "Get variable data from commongui_variables Table"
        n123 = Unbundle By Name(w319) -> ("PlotterInfo (from DB).Devices"=w306:string[], "PlotterInfo (from DB).Variables"=w305:string[], "PlotterInfo (from DB).Display Names (for variables)"=w304:string[], "PlotterInfo (from DB).SQL Server Info"=w317:T14, "PlotterInfo (from DB).Variable Data ID"=w318:string)
        n124 = Concatenate Strings("SELECT * FROM commongui_variables WHERE id ='", w318, "'" ("string")) -> (w298:string)
        n125 = call "SQL Query.vi"("error in (no error)"=w323, "SQL Server Info"=w317, "Query"=w298) -> ("error out"=w322:errorcluster, "data"=w314:string[][])  [unwired: 7 in]
        n126 = Index Array(array=w314) -> (element=w307:string[])  [unwired: 2 in]
        n127 = Array Subset(array=w307, index=9, length=4) -> (w301:string[])
        n128 = Array Subset(array=w307, index=13, length=4) -> (w302:string[])
        n129 = Array Subset(array=w307, index=5, length=4) -> (w303:string[])
        n130 = Build Array(w306, w305, w304, w303, w302, w301) -> (w300:string[][])
        n131 = Transpose 2D Array(2D array=w300) -> (transposed array=w299:string[][])
        n132 = for {
          tunnel: w299 -> [w327] mode=indexing
          tunnel: [w327] -> w320 mode=indexing if=w326
          n133 = call-poly <userlib>:"Filter 1D Array__ogtk.vi"("items to filter"="", "array"=w327) -> ("filtered array"=w329:string[])  [unwired: 4 in, 1 out]
          n134 = Empty Array?(array=w329) -> (empty?=w328:bool)
          n135 = Not(x=w328) -> (.not. x?=w326:bool)
        }
        n136 = Bundle By Name(cluster=w319, "PlotterInfo (from DB).Variable display info"=w320) -> (w321:T12)
        n137 = call <vilib>:"Add State(s) to Queue__jki_lib_state_machine.vi"("State(s) in (\"\")"=w325) -> ("States Out"=w324:string)  [unwired: 14 in]
      }
      frame "Data: Initialize Conections" {
        n138 = Unbundle By Name(w340) -> ("Data.Simulate"=w341:bool, "PlotterInfo (from DB).Variable display info"=w338:string[][], "Subscribe commands"=w334:string[])
        n139 = flat-sequence {
          tunnel: w341 -> [w349]
          tunnel: w338 -> [w348]
          tunnel: w337 -> [w347]
          tunnel: [w346] -> w336
          tunnel: w334 -> [w344]
          tunnel: [w345] -> w333
          tunnel: [w366] -> w335
          tunnel: w333 -> [w366]
          tunnel: w332 -> [w365]
          tunnel: [TRUE ("Data.Init")] -> w331
          frame #0 {
            n140 = case shown="False" w349 {
              tunnel: w348 -> [w359 _]
              tunnel: [w350 w363] -> w346
              tunnel: w347 -> [w351 w363]
              tunnel: [w352 w362] -> w345
              tunnel: w344 -> [_ w362]
              frame False {
                # "Generate Subscription Information"
                n141 = call "preset SQL Queries.vi"("error in (no error)"=w351, "Preset Query"=Preset_Query_Enum."Get all devices basic properties") -> ("error out"=w350:errorcluster, "data"=w357:string[][])  [unwired: 7 in, 1 out]
                "Device Infor from Database" <- w357
                n142 = Build Array (concatenate)(string[][] [["device", "variablename", "defaultvalue", "startvalue", "endvalue"]] ("Data"), w359) -> (w360:string[][])
                "appended array" <- w360
                n143 = call "scan data to receive to subscribe commands.vi"("ScanData to receive"=w360) -> ("devices"=w356:string[], "Subscribe commands"=w355:string[])  [unwired: 8 in, 1 out]
                n144 = call "get info from core device data.vi"("devices to get data from"=w356, "All Devices Core Info"=w357) -> ("Ports"=w354:string[], "IP Addresses"=w353:string[])  [unwired: 2 in]
                n145 = call "build tcp initialize message for process vis.vi"("IP Addresses"=w353, "Ports"=w354, "Subscribe commands"=w355) -> ("subscribe messages\nfor process vis"=w352:string[])  [unwired: 8 in]
                "Subscribe commands" <- w352
              }
              frame True {
                # "Simulate Mode"
              }
            }
          }
          frame #1 {
            n146 = Set Occurrence(w365) -> ()
          }
        }
        n147 = Bundle By Name(cluster=w340, "Subscribe commands"=w335, "Data.Init"=w331) -> (w339:T12)
        n148 = call <vilib>:"Add State(s) to Queue__jki_lib_state_machine.vi"("State(s) in (\"\")"=w343) -> ("States Out"=w342:string)  [unwired: 14 in]
      }
      frame "---------- UI ----------" {
        # "Do not put any code in this frame.\n(It is a separator no-op. You can make a copy of this frame to create a new UI frame)"
        n149 = call <vilib>:"Add State(s) to Queue__jki_lib_state_machine.vi"("State(s) in (\"\")"=w370) -> ("States Out"=w369:string)  [unwired: 14 in]
      }
      frame "UI: Initialize" {
        # "Initialize the User Interface, here.\n(this is called automatically, by the Macro: Init)"
        n150 = Unbundle By Name(w371) -> ("GUI controls.Stop"=w376:bool, "GUI controls.Tab Control"=w377:enum32{"Home", "Settings", "Plot", "Save"}, "GUI controls.Settings"=w375:bool, "GUI controls.Home"=w374:bool, "GUI controls.Plot"=w373:bool, "Data.Selected Variables"=w372:string[][])  [unwired: 2 out]
        n151 = property on="Stop" class="Bool"("Visible"=w376) -> ()  [unwired: 2 in, 2 out]
        n152 = property on="Database Variable List" class="MCListbox (strict)"("ItemNames"=w372) -> ()  [unwired: 2 in, 2 out]
        n153 = property on="Settings" class="Bool (strict)"("Value"=w375) -> ()  [unwired: 2 in, 2 out]
        n154 = property on="Plot" class="Bool (strict)"("Value"=w373) -> ()  [unwired: 2 in, 2 out]
        n155 = property on="Home" class="Bool (strict)"("Value"=w374) -> ()  [unwired: 2 in, 2 out]
        n156 = property on="Tab Control" class="TabCtl (strict)"("Value"=w377) -> ()  [unwired: 2 in, 2 out]
        n157 = call <vilib>:"Add State(s) to Queue__jki_lib_state_machine.vi"("State(s) in (\"\")"=w380) -> ("States Out"=w379:string)  [unwired: 14 in]
      }
      frame "UI: Cursor Set" {
        # "Argument"
        # "Set and Unset Cursor Busy.\n(Usage: \"UI: Cursor Set >> Busy|Idle\")"
        n158 = case shown="\"Idle\", Default" w381 {
          tunnel: w383 -> [w388 w390]
          tunnel: [w387 w389] -> w382
          frame "Idle", Default {
            n159 = call <vilib>:"Unset Busy.vi"("error in (no error)"=w388) -> ("error out"=w387:errorcluster)  [unwired: 10 in]
          }
          frame "Busy" {
            n160 = call <vilib>:"Set Busy.vi"("error in (no error)"=w390) -> ("error out"=w389:errorcluster)  [unwired: 9 in, 1 out]
          }
        }
        n161 = call <vilib>:"Add State(s) to Queue__jki_lib_state_machine.vi"("State(s) in (\"\")"=w386) -> ("States Out"=w385:string)  [unwired: 14 in]
      }
      frame "UI: Front Panel State" {
        # "Argument"
        # "Set Front Panel Open or Closed\n(Usage: \"UI: Front Panel State >> Open|Close\")"
        n162 = Unbundle By Name(w393) -> ("Core.Current VI Reference"=w392:refnum<vi>)
        n163 = case shown="\"Open\", Default" w391 {
          tunnel: w395 -> [w401 w414]
          tunnel: [w403 w415] -> w394
          tunnel: w392 -> [w402 w412]
          frame "Open", Default {
            n164 = property class="VI"(reference=w402, error in=w401) -> (reference out=w399:refnum<vi>, error out=w400:errorcluster, "Front Panel.Open"=w398:bool)
            n165 = case shown="True" w398 {
              tunnel: [w406 w409] -> w403
              tunnel: w400 -> [w405 w409]
              tunnel: w399 -> [w404 _]
              frame False {
                n166 = invoke class="VI" method="FP.Open"(reference=w404, error in=w405, "Activate"=TRUE, "State"=T6."Standard") -> (error out=w406:errorcluster)  [unwired: 1 in, 4 out]
              }
              frame True {
              }
            }
          }
          frame "Close" {
            n167 = property class="VI"(reference=w412, error in=w414) -> (reference out=w411:refnum<vi>, error out=w413:errorcluster, "Front Panel.Open"=w410:bool)
            n168 = case shown="True" w410 {
              tunnel: [w416 w419] -> w415
              tunnel: w413 -> [w416 w418]
              tunnel: w411 -> [_ w417]
              frame False {
              }
              frame True {
                n169 = invoke class="VI" method="FP.Close"(reference=w417, error in=w418) -> (error out=w419:errorcluster)  [unwired: 1 in, 2 out]
              }
            }
          }
        }
        n170 = call <vilib>:"Add State(s) to Queue__jki_lib_state_machine.vi"("State(s) in (\"\")"=w397) -> ("States Out"=w396:string)  [unwired: 14 in]
      }
      frame "---------- Macro ----------" {
        # "Do not put any code in this frame.\n(It is a separator no-op. You can make a copy of this frame to create a new Macro frame)"
        n171 = call <vilib>:"Add State(s) to Queue__jki_lib_state_machine.vi"("State(s) in (\"\")"=w423) -> ("States Out"=w422:string)  [unwired: 14 in]
      }
      frame "Macro: Initialize" {
        # "Initialization Macro\n(This is called once, when the VI starts)"
        n172 = disable-structure shown="Enabled" {
          disable-tunnel: w427 -> [w432 w433]
          disable-tunnel: [w431 w433] -> w426
          frame Enabled {
            n173 = call <userlib>:"Fit VI window to Largest Dec__ogtk.vi"("error in (no error)"=w432, "border spacing (2 px)"=0) -> ("error out"=w431:errorcluster)  [unwired: 4 in, 1 out]
          }
          frame Disabled {
          }
        }
        n174 = call <vilib>:"Add State(s) to Queue__jki_lib_state_machine.vi"("State(s) in Front (\"\")"="Data: Initialize\nInitialize Core Data\nUI: Initialize\nUI: Front Panel State >> Open\nData: Read Database\nData: Read Database 2\nData: Initialize Conections\nAction: Select All Data", "State(s) in (\"\")"=w429) -> ("States Out"=w428:string)  [unwired: 13 in]
      }
      frame "Macro: Exit" {
        w434 = FALSE ("create if not found? (T)")
        # "Exit Macro\n(This is called once, when the VI exits)"
        n175 = Unbundle By Name(w446) -> ("Core.Close Panel on Exit?"=w445:bool)
        n176 = Select(t="UI: Front Panel State >> Close", s=w445, f="") -> (s? t:f=w442:string)
        n177 = call <vilib>:"Add State(s) to Queue__jki_lib_state_machine.vi"("State(s) in (\"\")"=w442, "State(s) at Back (\"\")"="Data: Cleanup\nExit") -> ("States Out"=w440:string)  [unwired: 13 in]
        n178 = Obtain Queue(max queue size (-1, unlimited)=1, name (unnamed)="DeviceStopqueue", element data type=w434, create if not found? (T)=w434) -> (queue out=w439:refnum<queue>, error out=w435:errorcluster)  [unwired: 1 in, 1 out]
        n179 = Lossy Enqueue Element(queue=w439, element=TRUE, error in (no error)=w435) -> ()  [unwired: 4 out]
        n180 = call <vilib>:"Add State(s) to Queue__jki_lib_state_machine.vi"("State(s) in Front (\"\")"=w440, "State(s) in (\"\")"=w449) -> ("States Out"=w448:string)  [unwired: 13 in]
      }
      frame "---------- Action ----------" {
        # "Template Separator\n(You can make a copy of, or modify, this frame)"
        n181 = call <vilib>:"Add State(s) to Queue__jki_lib_state_machine.vi"("State(s) in (\"\")"=w453) -> ("States Out"=w452:string)  [unwired: 14 in]
      }
      frame "Action: Start Plotting" {
        n182 = property on="Stop" class="Bool"("Visible"=TRUE) -> ()  [unwired: 2 in, 2 out]
        n183 = Unbundle By Name(w459) -> ("Data.Selected Variables"=w463:string[][])
        n184 = Array Size(array=w463) -> (size(s)=w464:i32[])
        n185 = Index Array(array=w464) -> (element=w461:i32)  [unwired: 1 in]
        n186 = Add(x=w461, y=w461) -> (x+y=w460:i32)
        n187 = Initialize Array(cluster{timestamp[], dbl[]} {[], []} ("Graph i"), w460) -> (w454:cluster{timestamp[], dbl[]}[])
        n188 = Bundle By Name(cluster=w459, "Data.No of Selected Variables"=w460, "Graph.Graph Data Long"=w454, "Graph.Graph Data Short"=w454) -> (w458:T12)
        n189 = call <vilib>:"Add State(s) to Queue__jki_lib_state_machine.vi"("State(s) in (\"\")"=w457) -> ("States Out"=w456:string)  [unwired: 14 in]
      }
      frame "Action: Plot Data" {
        # "Timer calculations:\nPlot 1 data updates \nafter every 30 seconds"
        # "#TODO Hide the RHS scales on the long term plot and the\nLHS scales on the short term plot\nBring both plots closer."
        # "This case is used for long term and short term data plotting"
        n190 = Unbundle By Name(w484) -> ("Graph.ms timer value"=w471:u32, "Graph.Graph Data Long"=w482:T15, "Data.Data"=w480:dbl[], "Data.Selected Variables"=w466:string[][], "Data.Currently selected items"=w486:i32[], "Graph.Long term plot"=w467:refnum<vi>, "Graph.Graph Data Short"=w468:T15)
        n191 = First Call?() -> (First Call?: T/F=w476:bool)
        n192 = call <userlib>:"Tick Count (ms)__ogtk.vi"() -> ("millisecond timer value"=w472:u32)  [unwired: 10 in, 1 out]
        n193 = Not(x=w476) -> (.not. x?=w474:bool)
        n194 = Subtract(x=w472, y=w471) -> (x-y=w477:u32)
        n195 = call "Plot.vi"("dev-Var data"=w480, "Selected Variables"=w466, "Currently selected items"=w486) -> ("Plot Data"=w479:dbl[])  [unwired: 12 in]
        n196 = Greater Or Equal?(x=w477, y=u32 30000 ("min time between updates")) -> (x >= y?=w475:bool)
        n197 = And(x=w475, y=w474) -> (x .and. y?=w473:bool)
        n198 = call "Graph Properties Runtime.vi"("Long Term Graph"=w467, "Selected Variables"=w466, "Plot Data"=w479) -> ()  [unwired: 12 in, 1 out]
        n199 = case shown="True" w473 {
          tunnel: "Clear Graph" -> [_ w503]
          tunnel: w482 -> [w497 w501]
          tunnel: [w497 w500] -> w481
          tunnel: w479 -> [_ w499]
          tunnel: w472 -> [_ w498]
          tunnel: w471 -> [w496 _]
          tunnel: [w496 w498] -> w470
          frame False {
          }
          frame True {
            n200 = call "Long Term PLot.vi"("Graph Data"=w501, "Plot Data"=w499, "Clear Graph"=w503, "Max Number of Datapoints"=2000.0) -> ("Graph Data 2"=w500:T15)  [unwired: 11 in]
            "Long Term Plot" <- w500
          }
        }
        n201 = case shown="True" w474 {
          tunnel: "Clear Graph" -> [_ w495]
          tunnel: w468 -> [w490 w493]
          tunnel: w479 -> [_ w492]
          tunnel: [w490 w491] -> w469
          frame False {
          }
          frame True {
            n202 = call "Long Term PLot.vi"("Graph Data"=w493, "Plot Data"=w492, "Clear Graph"=w495, "Max Number of Datapoints"=500.0) -> ("Graph Data 2"=w491:T15)  [unwired: 11 in]
            "short Term Plot" <- w491
          }
        }
        n203 = Bundle By Name(cluster=w484, "Graph.ms timer value"=w470, "Graph.Graph Data Long"=w481, "Graph.Graph Data Short"=w469) -> (w485:T12)
        n204 = call <vilib>:"Add State(s) to Queue__jki_lib_state_machine.vi"("State(s) in (\"\")"=w489) -> ("States Out"=w488:string)  [unwired: 14 in]
      }
      frame "Action: Collect Data" {
        # "Collect Data from TCP port/ Simulated data"
        n205 = Unbundle By Name(w509) -> ("Data.Selected Variables"=w506:string[][], "Data.Simulate"=w512:bool, "PlotterInfo (from DB).Device space Variable"=w504:string[])
        n206 = case shown="False" w512 {
          tunnel: w511 -> [w527 w545]
          tunnel: [w527 w545] -> w510
          tunnel: [w516 w541] -> w507
          tunnel: w506 -> [w524 w543]
          tunnel: w505 -> [w525 _]
          tunnel: w504 -> [w520 _]
          frame False {
            (unwired) dbl[] []
            # "Data from TCP port"
            n207 = Preview Queue Element(queue=w525, timeout in ms (-1)=200) -> (element=w523:string[][])  [unwired: 1 in, 3 out]
            "tcp Data" <- w523
            n208 = Index Array(array=w523, index (row) #1=0 ("index (row)"), index (row) #2=1 ("disabled index (col)")) -> (element #1=w521:string[], element #2=w518:string[])  [unwired: 2 in]
            "channels" <- w521
            "chnl data" <- w518
            n209 = for {
              tunnel: w521 -> [w540]
              tunnel: w520 -> [w539] mode=indexing
              tunnel: [w538] -> w519 mode=indexing
              n210 = Search 1D Array(1D array=w540, element=w539) -> (index of element=w538:i32)  [unwired: 1 in]
            }
            n211 = for {
              tunnel: w518 -> [w529] mode=indexing
              tunnel: [w528] -> w517 mode=indexing
              n212 = Fract/Exp String To Number(string=w529) -> (number=w528:dbl)  [unwired: 3 in, 1 out]
            }
            n213 = for {
              tunnel: w519 -> [w531] mode=indexing
              tunnel: w517 -> [w532]
              tunnel: [w530] -> w516 mode=indexing
              n214 = Less Than 0?(x=w531) -> (x < 0?=w533:bool)
              n215 = case shown="False" w533 {
                tunnel: [w534 0.0] -> w530
                tunnel: w532 -> [w536 _]
                tunnel: w531 -> [w535 _]
                frame False {
                  n216 = Index Array(array=w536, index=w535) -> (element=w534:dbl)
                }
                frame True {
                }
              }
            }
            "Selected Variables" <- w524
          }
          frame True {
            # "Simulated Data"
            n217 = Index Array(array=w543, index (col)=3 ("disabled index (col)")) -> (element=w542:string[])  [unwired: 1 in]
            n218 = for {
              tunnel: w542 -> [w548] mode=indexing
              tunnel: [w546] -> w541 mode=indexing
              n219 = Fract/Exp String To Number(string=w548) -> (number=w547:dbl)  [unwired: 3 in, 1 out]
              n220 = Random Number (0-1)() -> (number: 0 to 1=w549:dbl)
              n221 = Add(x=w549, y=w547) -> (x+y=w546:dbl)
            }
          }
        }
        n222 = Bundle By Name(cluster=w509, "Data.Data"=w507) -> (w508:T12)
        n223 = call <vilib>:"Add State(s) to Queue__jki_lib_state_machine.vi"("State(s) in (\"\")"=w514) -> ("States Out"=w513:string)  [unwired: 14 in]
      }
      frame "Action: Select All Data" {
        # "Graph properties needs to set only once \nso coded here"
        # "Select variables from configuration file"
        n224 = Unbundle By Name(w563) -> ("PlotterInfo (from DB).Variable display info"=w554:string[][], "Graph.Long term plot"=w562:refnum<vi>, "Graph.Short term plot"=w561:refnum<vi>)
        n225 = Array Size(array=w554) -> (size(s)=w558:i32[])
        n226 = Build Array(w562, w561) -> (w560:refnum<vi>[])
        n227 = Index Array(array=w558) -> (element=w557:i32)  [unwired: 1 in]
        n228 = Empty Array?(array=w554) -> (empty?=w550:bool)
        n229 = property on="Database Variable List" class="MCListbox (strict)"(error in=w551, "ItemNames"=w554) -> (error out=w552:errorcluster)  [unwired: 1 in, 1 out]
        n230 = case shown="False" w550 {
          tunnel: w560 -> [w572 _]
          tunnel: [w571 w573] -> w559
          tunnel: [w570 _] -> w556
          tunnel: w551 -> [w569 w573]
          tunnel: w554 -> [w568 _]
          frame False {
            n231 = call "Set Graph Properties.vi"("error out 2"=w569, "Selected Variables"=w568, "Reference Array"=w572) -> ("error out"=w571:errorcluster, "Legend rows"=w570:i32)  [unwired: 7 in]
          }
          frame True {
          }
        }
        n232 = for {
          N: w557 -> [_]
          tunnel: [w574] -> w564 mode=indexing
          i -> [w574]
        }
        n233 = control-ref of="Database Variable List"() -> (w553:refnum<vi>)
        n234 = Bundle By Name(cluster=w563, "Data.Currently selected items"=w564, "Data.Selected Variables"=w554, "Data.Legend Rows"=w556) -> (w565:T12)
        n235 = call "Listbox Properties.vi"("error in (no error)"=w552, "Configuration File Variable List 2"=w553) -> ()  [unwired: 9 in, 1 out]
        n236 = call <vilib>:"Add State(s) to Queue__jki_lib_state_machine.vi"("State(s) in Front (\"\")"="Action: Start Plotting" ("State(s) in Front (\"\")"), "State(s) in (\"\")"=w567) -> ("States Out"=w566:string)  [unwired: 13 in]
      }
    }
  }
  n237 = call "FGVDataStart.vi"("command"=enum16{"ini", "get", "set"}."ini") -> ()  [unwired: 9 in, 2 out]
  n238 = Obtain Queue(max queue size (-1, unlimited)=1, name (unnamed)="DeviceStopqueue", element data type=w23) -> (queue out=w25:refnum<queue>, error out=w21:errorcluster)  [unwired: 2 in, 1 out]
  n239 = Enqueue Element(queue=w25, element=w23, error in (no error)=w21) -> (queue out=w8:refnum<queue>, error out=w35:errorcluster)  [unwired: 1 in, 1 out]
  n240 = call "preset SQL Queries.vi"("error in (no error)"=w35, "Preset Query"=Preset_Query_Enum."GetLocalPortRange") -> ("error out"=w34:errorcluster, "data"=w33:string[][])  [unwired: 7 in, 1 out]
  n241 = call "reentrant tcp data get sub vi.vi"("tcp data event"=w28, "Ports"=w33, "error in (no error)"=w34, "tcpDataqueue"=w11, "Stopqueue"=w8, "subscribe messages for process vis"=w27) -> ("error out"=w26:errorcluster)  [unwired: 5 in]
  n242 = call <vilib>:"Clear Errors.vi"("error in (no error)"=w26) -> ("error out"=w13:errorcluster)  [unwired: 6 in]
  n243 = Merge Errors(w14, w13) -> (w12:errorcluster)
  n244 = call <vilib>:"Clear Errors.vi"("error in (no error)"=w12) -> ("error out"=w36:errorcluster)  [unwired: 6 in]
  n245 = Flush Queue(queue=w8, error in (no error)=w36) -> (queue out=w29:refnum<queue>, error out=w30:errorcluster)  [unwired: 1 out]
  n246 = Release Queue(queue=w29, force destroy? (F)=TRUE, error in (no error)=w30) -> (error out=w20:errorcluster)  [unwired: 2 out]
  n247 = Release Queue(queue=w11, error in (no error)=w20) -> (error out=w19:errorcluster)  [unwired: 1 in, 2 out]
  n248 = call <vilib>:"Clear Errors.vi"("error in (no error)"=w19) -> ("error out"=w9:errorcluster)  [unwired: 6 in]
  n249 = call "generateEvent.vi"("error in"=w9, "command"=enum16{"ini", "get", "close"}."close") -> ()  [unwired: 8 in, 2 out]
